vi "Load INI.vi"(8 "error in (no error)":errorcluster, 11 "HAL Editor in":refnum<class "HAL Editor.lvclass">) -> (0 "error out":errorcluster, 3 "HAL Editor out":refnum<class "HAL Editor.lvclass">)   [LabVIEW 2012, in "HAL Config.lvlib" / "HAL Editor.lvclass"]
uses:
  HAL Editor.lvclass
  build/ppl/lv-hal.lvlibp/HAL Manager/HAL Manager.lvclass
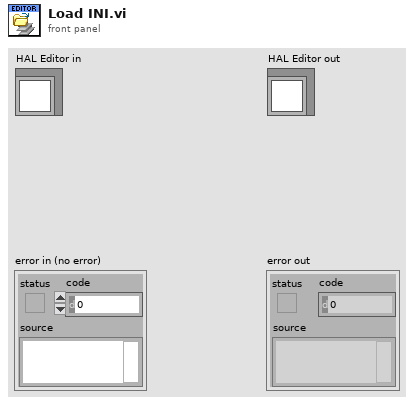
[diagram p1: front panel]
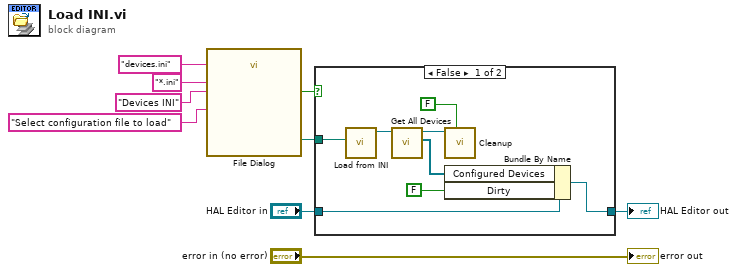
[diagram p0: block diagram]
diagram:
  n1 = call "File Dialog"("prompt"="Select configuration file to load" ("pattern label"), "default name"="devices.ini", "pattern (all files)"="*.ini", "pattern label"="Devices INI") -> ("selected path"=w3:path, "cancelled"=w4:bool)  [unwired: 8 in, 2 out]
  n2 = case shown="False" w4 {
    tunnel: "HAL Editor in" -> [w17 w18]
    tunnel: [w16 w18] -> w1
    tunnel: w3 -> [w14 _]
    frame False {
      n3 = call "Load from INI.vi"("INI Path"=w14) -> ("HAL Manager out"=w13:refnum<class "HAL Manager.lvclass">)  [unwired: 9 in, 1 out]
      n4 = call "Get All Devices.vi"("HAL Manager in"=w13) -> ("Devices"=w10:refnum<class "Device.lvclass">[], "HAL Manager out"=w12:refnum<class "HAL Manager.lvclass">)  [unwired: 8 in, 1 out]
      n5 = call "Cleanup.vi"("Cleanup Devices? (T)"=FALSE, "HAL Manager in"=w12) -> ()  [unwired: 9 in, 1 out]
      n6 = Bundle By Name(cluster=w17, "Configured Devices"=w10, "Dirty"=FALSE) -> (w16:refnum<class "HAL Editor.lvclass">)
    }
    frame True {
    }
  }
  "HAL Editor out" <- w1
  "error out" <- "error in (no error)"
